vi "ACT_Loop.vi"() -> ()   [LabVIEW 2023, in "Swerve AM_ACT.lvlib"]
uses:
  Swerve AM_ACT.lvlib
  RoboRIO Utilities/Global_STOP.vi
  ENUM_ACT_Action.ctl
  ENUM_ACT_State.ctl
  Global_CMD_ACT_Data In.vi
  Global_ACT_Data Out.vi
  Cluster_CMD_ACT_Data.ctl
  <vilib>/Rock Robotics/WPI/MotorControl/WPI_MotorControlType.ctl
  <vilib>/Rock Robotics/SystemInterfaces/DIO/FPGA_DIOPWMChannel.ctl
  <vilib>/Rock Robotics/WPI/PWM/WPI_PWMDeadband.ctl
  <vilib>/Rock Robotics/SystemInterfaces/DIO/FPGA_DIOChannel.ctl
  <vilib>/Rock Robotics/WPI/MotorControl/WPI_MotorControlDeviceRef.ctl
  <vilib>/Rock Robotics/WPI/ThirdParty/Phoenix-LabVIEW/Motor Controller/Controls/CTRE_Phoenix_MotorControl_NeutralMode.ctl
  Shared Code/TypeDefs/Cluster_FWD  REV Values.ctl
  Shared Code/TypeDefs/Cluster_Config SRX Motor Output.ctl
  Shared Code/TypeDefs/Cluster_PID Gains.ctl
  Shared Code/TypeDefs/Cluster_SRX SLOT PID Config.ctl
  Cluster_Config HW Values.ctl
  b5508d6c-c1cc-4273-80c5-2077d34e1483.vi
  5f725c2a-0ce1-4524-8967-e83b15fdce90.vi
  <vilib>/Rock Robotics/WPI/ThirdParty/Phoenix-LabVIEW/Motor Controller/Controls/CTRE_Phoenix_MotorControl_ControlMode.ctl
  Cluster_HW Output Values.ctl
  ENUM_CMD_Mode Select.ctl
  4f1f8321-3dc8-4b28-8619-20673fc77ec2.vi
  Cluster_System Output Data.ctl
  Cluster_Config System Values.ctl
  36677ea0-a1a5-47a3-bc56-4475cb7c281e.vi
  573e44c0-11f4-4bd9-ad56-904ec25dba75.vi
  e7494af9-f670-4352-9dfa-ae6ce50709ea.vi
  6201c2b1-dcd8-4430-86f1-9b4ee56c7753.vi
  Shared Code/TypeDefs/ENUM_Module Position.ctl
  t-shirt-robot/T-Shirt Robot LV 2020/roboRIO Code/Systems/SwerveDrive AM/Cluster_Config Specific Data.ctl
  t-shirt-robot/T-Shirt Robot LV 2020/roboRIO Code/Systems/SwerveDrive AM/Cluster_Config Specific HW Values.ctl
  Shared Code/TypeDefs/Dial_Compase heading unit circle CCW positive.ctl
  Shared Code/TypeDefs/Level_Velocity plus-minus 1.ctl
  Shared Code/TypeDefs/Cluster_Module Velocity-Direction-Rotations.ctl
  Shared Code/TypeDefs/Cluster_Swerve 4 Steer and Velocity.ctl
  Shared Code/TypeDefs/Cluster_Config_SwerveParam Drive.ctl
  Shared Code/TypeDefs/Cluster_Config_SwerveParam Steer.ctl
  Type Defs/Cluster_Length and Width.ctl
  Cluster_Config Steer HW Values.ctl
  t-shirt-robot/T-Shirt Robot LV 2020/roboRIO Code/Systems/SwerveDrive AM/Cluster_Config Drive HW Values.ctl
  Shared Code/TypeDefs/Cluster_X-Y.ctl
  Shared Code/TypeDefs/Cluster_CMD_Direction Data.ctl
  PigeonIMU/Global_SEN_Data Out.vi
  PigeonIMU/PigeonIMU_SEN_ts.lvlib
  089052c0-d540-4a78-a5cc-aeb70dbb496b.vi
  f366bc00-a3dd-4e55-84f0-76161afbb392.vi
  6826157a-0860-4dcc-86dd-81ceae711a6e.vi
  Shared Code/TypeDefs/Cluster_Config Spark Max Motor Output.ctl
  <vilib>/Rock Robotics/WPI/ThirdParty/REV Robotics/REVLib/Typedef/Spark MAX Idle Mode.ctl
  Shared Code/TypeDefs/Cluster_High-Low.ctl
  Shared Code/TypeDefs/Cluster_Spark MAX SLOT PID Config.ctl
  Shared Code/TypeDefs/Cluster_SW PID Config.ctl
  cae143b2-6fb3-4693-aed3-53517d8ac0dc.vi
  c90b907c-c448-477a-a93b-8b17a70bee0e.vi
  Shared Code/TypeDefs/Cluster_SparkMax Smart Motion Parameters.ctl
  Shared Code/TypeDefs/Cluster_SRX Motion Magic Parameters.ctl
panel:
  in  "Config Drive":T1={"Drive HW Ver"=0, "SparkMax Output"={"Idle Mode"=enum."Coast", "Ramp Rate (S)"=0.0}, "Slot 0 CL"={"Gains"={"P"=0.1, "I"=0.0, "D"=0.0, "F"=0.0}, "I Zone"=0.0, "Peak Out -1 0 1"={"High"=0.0, "Low"=0.0}, "Max I Accu"=0.0}, "Slot 0 SM"={"Max Velocity"=1.0, "Max Acceleration"=0.0, "Allowed CL Error"=0.0, "Min Velocity Output"=0.0}} {"Slot 0 CL"."Gains"."F" format="%#.8f"; "Slot 0 CL"."Gains"."D" format="%#.8f"; "Slot 0 CL"."Gains"."I" format="%#.8f"; "Slot 0 CL"."Gains"."P" format="%#.8f"; "Slot 0 CL"."Peak Out -1 0 1"."Low" format="%#.8f"; "Slot 0 CL"."Peak Out -1 0 1"."High" format="%#.8f"}
  in  "Config Steer":T8={"Steer HW Ver"=0, "SRX Output"={"Neutral"=enum."Override to Coast", "Max"={"FWD"=1.0, "REV"=-1.0}, "Min"={"FWD"=0.0, "REV"=0.0}, "OL Ramp Rate (S)"=0.0, "Dead Band"=0.0, "CL Ramp Rate (S)"=0.0}, "Slot 0 CL"={"Gains"={"P"=1.0, "I"=0.01, "D"=0.0, "F"=0.0}, "Error Allowed"=0.0, "I Zone"=10000.0, "Peak Out 0-1"=1.0, "Max I Accu"=-1000.0}, "Slot 0 MM"={"Cruise Velocity"=5000, "Acceleration"=5000}} {"Slot 0 CL"."Gains"."F" format="%#.8f"; "Slot 0 CL"."Gains"."D" format="%#.8f"; "Slot 0 CL"."Gains"."I" format="%#.8f"; "Slot 0 CL"."Gains"."P" format="%#.8f"; "SRX Output"."Min"."REV" format="%.2f"; "SRX Output"."Min"."FWD" format="%.2f"; "SRX Output"."Max"."REV" format="%.2f"; "SRX Output"."Max"."FWD" format="%.2f"}
  in  "HW Specific Config":T14={"Specific HW Ver"=0, "Specific Data"=[{"Motor Pos"=enum."Left-Front", "CAN Bus"="", "Drive ID"=0, "Drive Invert"=FALSE, "Steer ID"=0, "Steer Invert"=FALSE, "Encoder Start Value"=0.0}, {"Motor Pos"=enum."Right-Front", "CAN Bus"="", "Drive ID"=0, "Drive Invert"=FALSE, "Steer ID"=0, "Steer Invert"=FALSE, "Encoder Start Value"=0.0}, {"Motor Pos"=enum."Right-Back", "CAN Bus"="", "Drive ID"=0, "Drive Invert"=FALSE, "Steer ID"=0, "Steer Invert"=FALSE, "Encoder Start Value"=0.0}, {"Motor Pos"=enum."Left-Back", "CAN Bus"="", "Drive ID"=0, "Drive Invert"=FALSE, "Steer ID"=0, "Steer Invert"=FALSE, "Encoder Start Value"=0.0}]}
  in  "CMD Override":enum32{"None", "Mode 2", "Mode 1", "STOP"}(tab)
  in  "Mode 2 Data":dbl(slide) scale=-0.2..0.2
  in  "Mode 1 Data":i32
  in  "GO":bool
  out "Current Time":timestamp
  in  "System Config":T17={"System Ver"=0, "Auto Angle PID"={"Gains"={"P"=0.1, "I"=0.0, "D"=0.0, "F"=0.0}, "Error Allowed"={"High"=0.0, "Low"=0.0}, "I Zone"={"High"=0.0, "Low"=0.0}, "Peak Out 0-1"={"High"=0.0, "Low"=0.0}, "Max I Accu"={"High"=0.0, "Low"=0.0}}, "Frame"={"Length"=33.0, "Width"=18.0}, "DriveTrain"={"CPR"=14.0, "RevMotor/Wheel"=6.67, "Wheel Diameter (in)"=4.0}, "Speed Full Scale"=5000.0, "Steer Data"={"CPR"=1024.0}} {"Auto Angle PID"."Max I Accu"."Low" format="%#.8f"; "Auto Angle PID"."Max I Accu"."High" format="%#.8f"; "Auto Angle PID"."Gains"."F" format="%#.8f"; "Auto Angle PID"."Gains"."D" format="%#.8f"; "Auto Angle PID"."Gains"."I" format="%#.8f"; "Auto Angle PID"."Gains"."P" format="%#.8f"; "Auto Angle PID"."Error Allowed"."Low" format="%#.8f"; "Auto Angle PID"."Error Allowed"."High" format="%#.8f"; "Auto Angle PID"."I Zone"."Low" format="%#.8f"; "Auto Angle PID"."I Zone"."High" format="%#.8f"; "Auto Angle PID"."Peak Out 0-1"."Low" format="%#.8f"; "Auto Angle PID"."Peak Out 0-1"."High" format="%#.8f"}
  out "System Config":T22
  out "Sensor Read time":dbl format="%.3g"
  out "HW Output":T23 {"Swerve Read"."Back Right"."Angle" scale format="%.3f"; "Swerve Read"."Back Right"."Velocity" scale=-1.0..1.0 scale format="%.1f"; "Swerve Read"."Back Left"."Angle" scale format="%.3f"; "Swerve Read"."Back Left"."Velocity" scale=-1.0..1.0 scale format="%.1f"; "Swerve Read"."Front Left"."Angle" scale format="%.3f"; "Swerve Read"."Front Left"."Velocity" scale=-1.0..1.0 scale format="%.1f"; "Swerve Read"."Front Right"."Angle" scale format="%.3f"; "Swerve Read"."Front Right"."Velocity" scale=-1.0..1.0 scale format="%.1f"; "Pigeon Heading" scale format="%.3f"}
  in  "Read Saved Config":bool
  in  "Update Config":bool
  out "CMD":T28 {"Target Auto Angle" scale format="%.3f"; "Direction"."Rotate(Yaw) CCW 1 CW -1" scale=1.0..-1.0; "Direction"."Traverse"."Angle" scale format="%.3f"; "Direction"."Traverse"."Velocity" scale=-1.0..1.0 scale format="%.1f"}
  out "Cycle Time (S)":dbl format="%.3g"
  # "STOP"
  # "\"Front\" of Robot"
  # "Right Hand Rule"
  # "X"
  # "+CCW"
  # "Y"
  # "(0,0)"
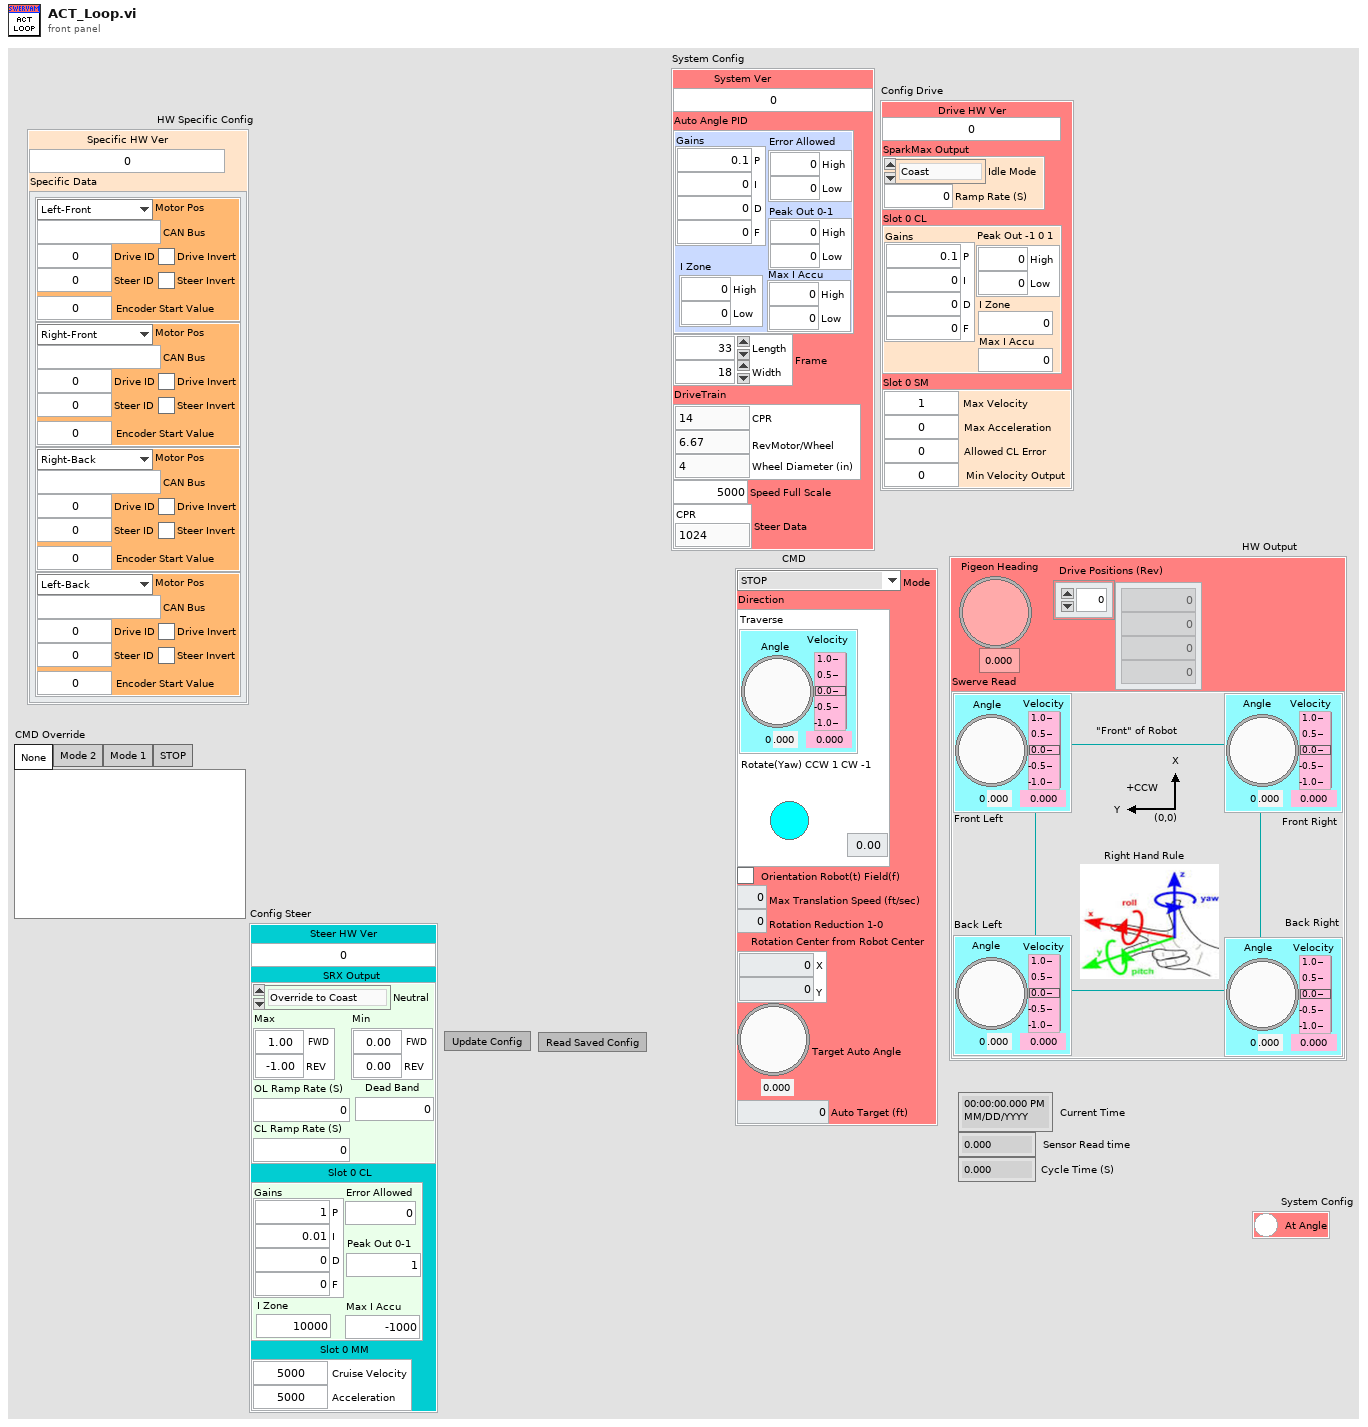
[diagram p1: front panel]
types:
  T1 = typedef "Swerve AM_ACT.lvlib/Cluster_Config Drive HW Values.ctl" = cluster{"Drive HW Ver":u64, "SparkMax Output":T2, "Slot 0 CL":T4, "Slot 0 SM":T7}
  T2 = typedef "Cluster_Config Spark Max Motor Output.ctl" = cluster{"Idle Mode":T3, "Ramp Rate (S)":dbl}
  T3 = typedef "Spark MAX Idle Mode.ctl" = enum16{"Coast", "Brake"}
  T4 = typedef "Cluster_Spark MAX SLOT PID Config.ctl" = cluster{"Gains":T5, "I Zone":dbl, "Peak Out -1 0 1":T6, "Max I Accu":dbl}
  T5 = typedef "Cluster_PID Gains.ctl" = cluster{"P":dbl, "I":dbl, "D":dbl, "F":dbl}
  T6 = typedef "Cluster_High-Low.ctl" = cluster{"High":dbl, "Low":dbl}
  T7 = typedef "Cluster_SparkMax Smart Motion Parameters.ctl" = cluster{"Max Velocity":dbl, "Max Acceleration":dbl, "Allowed CL Error":dbl, "Min Velocity Output":dbl}
  T8 = typedef "Swerve AM_ACT.lvlib/Cluster_Config Steer HW Values.ctl" = cluster{"Steer HW Ver":u64, "SRX Output":T9, "Slot 0 CL":T12, "Slot 0 MM":T13}
  T9 = typedef "Cluster_Config SRX Motor Output.ctl" = cluster{"Neutral":T10, "Max":T11, "Min":T11, "OL Ramp Rate (S)":dbl, "Dead Band":dbl, "CL Ramp Rate (S)":dbl}
  T10 = typedef "CTRE_Phoenix_MotorControl_NeutralMode.ctl" = enum8{"EEPROMSetting", "Override to Coast", "Override to Brake"}
  T11 = typedef "Cluster_FWD  REV Values.ctl" = cluster{"FWD":dbl, "REV":dbl}
  T12 = typedef "Cluster_SRX SLOT PID Config.ctl" = cluster{"Gains":T5, "Error Allowed":dbl, "I Zone":dbl, "Peak Out 0-1":dbl, "Max I Accu":dbl}
  T13 = typedef "Cluster_SRX Motion Magic Parameters.ctl" = cluster{"Cruise Velocity":i32, "Acceleration":i32}
  T14 = typedef "Swerve AM_ACT.lvlib/Cluster_Config Specific HW Values.ctl" = cluster{"Specific HW Ver":u64, "Specific Data":T15[]}
  T15 = typedef "Swerve AM_ACT.lvlib/Cluster_Config Specific Data.ctl" = cluster{"Motor Pos":T16, "CAN Bus":string, "Drive ID":u8, "Drive Invert":bool, "Steer ID":u8, "Steer Invert":bool, "Encoder Start Value":dbl}
  T16 = typedef "ENUM_Module Position.ctl" = enum16{"Left-Front", "Right-Front", "Left-Back", "Right-Back"}
  T17 = typedef "Swerve AM_ACT.lvlib/Cluster_Config System Values.ctl" = cluster{"System Ver":u64, "Auto Angle PID":T18, "Frame":T19, "DriveTrain":T20, "Speed Full Scale":dbl, "Steer Data":T21}
  T18 = typedef "Cluster_SW PID Config.ctl" = cluster{"Gains":T5, "Error Allowed":T6, "I Zone":T6, "Peak Out 0-1":T6, "Max I Accu":T6}
  T19 = typedef "Cluster_Length and Width.ctl" = cluster{"Length":dbl, "Width":dbl}
  T20 = typedef "Cluster_Config_SwerveParam Drive.ctl" = cluster{"CPR":dbl, "RevMotor/Wheel":dbl, "Wheel Diameter (in)":dbl}
  T21 = typedef "Cluster_Config_SwerveParam Steer.ctl" = cluster{"CPR":dbl}
  T22 = typedef "Swerve AM_ACT.lvlib/Cluster_System Output Data.ctl" = cluster{"At Angle":bool}
  T23 = typedef "Swerve AM_ACT.lvlib/Cluster_HW Output Values.ctl" = cluster{"Pigeon Heading":T24, "Swerve Read":T25, "Drive Positions (Rev)":dbl[]}
  T24 = typedef "Dial_Compase heading unit circle CCW positive.ctl" = dbl
  T25 = typedef "Cluster_Swerve 4 Steer and Velocity.ctl" = cluster{"Front Right":T26, "Front Left":T26, "Back Left":T26, "Back Right":T26}
  T26 = typedef "Cluster_Module Velocity-Direction-Rotations.ctl" = cluster{"Velocity":T27, "Angle":T24, "Rotations Count":dbl}
  T27 = typedef "Level_Velocity plus-minus 1.ctl" = dbl
  T28 = typedef "Swerve AM_ACT.lvlib/Cluster_CMD_ACT_Data.ctl" = cluster{"Mode":T29, "Direction":T30, "Orientation Robot(t) Field(f)":bool, "Max Translation Speed (ft/sec)":dbl, "Rotation Reduction 1-0":dbl, "Rotation Center from Robot Center":T31, "Target Auto Angle":T24, "Auto Target (ft)":dbl}
  T29 = typedef "Swerve AM_ACT.lvlib/ENUM_CMD_Mode Select.ctl" = enum16{"STOP", "Move", "Turret Manual", "Trans Manual Angle Auto", "Turret Auto Angle"}
  T30 = typedef "Cluster_CMD_Direction Data.ctl" = cluster{"Traverse":T26, "Rotate(Yaw) CCW 1 CW -1":dbl}
  T31 = typedef "Cluster_X-Y.ctl" = cluster{"X":dbl, "Y":dbl}
  T32 = typedef "Swerve AM_ACT.lvlib/ENUM_ACT_Action.ctl" = enum16{"No Action", "Reset Time", "Reset All", "Config HW File Read", "Config HW File Save", "Config SW File Read", "Config SW File Save", "Config From FP", "Config HW All Get", "Config HW Set Steer", "Open HW Only", "Control FX Stop", "Control FX Mode 1", "Control FX Mode 2", "Set Robot Start Position", "Config HW Set Drive"}
  T33 = typedef "WPI_MotorControlDeviceRef.ctl" = cluster{"DeviceStatus":errorcluster, "Type":T34, "PWM":cluster{"PWM Channel":T35, "DeadBand":T36}, "CAN":cluster{"Device Number":u8, "SetOutput VI Ref":variant, "GetOutput VI Ref":variant, "Enable VI Ref":variant, "Disable VI Ref":variant, "Data":variant}, "Invert":bool, "DIO PWM":cluster{"PWM \"Enable\" Channel":T35, "DIOChannel":T37, "PWM Rate":dbl}}
  T34 = typedef "WPI_MotorControlType.ctl" = enum16{"PWM", "CAN", "DIO PWM"}
  T35 = typedef "FPGA_DIOPWMChannel.ctl" = enum8{"PWM 0", "PWM 1", "PWM 2", "PWM 3", "PWM 4", "PWM 5", "PWM 6", "PWM 7", "PWM 8", "PWM 9", "PWM MXP 0", "PWM MXP 1", "PWM MXP 2", "PWM MXP 3", "PWM MXP 4", "PWM MXP 5", "PWM MXP 6", "PWM MXP 7", "PWM MXP 8", "PWM MXP 9", "Invalid"}
  T36 = typedef "WPI_PWMDeadband.ctl" = cluster{"Name":string, "maxPositivePwm":i32, "minPositivePwm":i32, "centerPwm":i32, "maxNegativePwm":i32, "minNegativePwm":i32, "angularRange":u16}
  T37 = typedef "FPGA_DIOChannel.ctl" = enum8{"DIO 0", "DIO 1", "DIO 2", "DIO 3", "DIO 4", "DIO 5", "DIO 6", "DIO 7", "DIO 8", "DIO 9", "DIO MXP 0", "DIO MXP 1", "DIO MXP 2", "DIO MXP 3", "DIO MXP 4", "DIO MXP 5", "DIO MXP 6", "DIO MXP 7", "DIO MXP 8", "DIO MXP 9", "DIO MXP 10", "DIO MXP 11", "DIO MXP 12", "DIO MXP 13", "DIO MXP 14", "DIO MXP 15", "SPI Port CS1", "SPI Port CS2", "SPI Port CS3", "SPI Port MISO", "SPI Port MOSI", "Invalid"}
  T38 = typedef "Swerve AM_ACT.lvlib/Cluster_Config HW Values.ctl" = cluster{"Drive":T1, "Steer":T8}
  T39 = typedef "CTRE_Phoenix_MotorControl_ControlMode.ctl" = u16
  T40 = typedef "Swerve AM_ACT.lvlib/ENUM_ACT_State.ctl" = enum16{"Startup", "Configuring", "Stopping", "Moving Mode 1", "Moving Mode 2", "Shutdown", "Initializing HW"}
  T41 = cluster{"Motor List":T16[], "Team Folder":path, "FX Ref":T33, "Steer Refs":T33[], "Drive Refs":T33[], "State":T40, "Previous State":T40, "Current Time":timestamp, "Previous Time":timestamp, "Start Time":timestamp, "Target Time (ms)":u32, "Cycle Time(S)":dbl, "Update Display":bool, "ACT Input":T28, "HW All Config":T38, "Config System":T17, "Max # Of Config Tries":i32, "HW Out":T23, "System Output":T22, "CAN Timeout":u32, "FX Mode":T39, "FX Set Value":dbl, "Config HW Specific":T14, "Swerve Set":T25, "New Cmd":bool, "Config HW Steer":T8, "Config HW Drive":T1}
  T42 = enum16{"No Action", "Reset Time", "Reset All", "Config HW File Read", "Config HW File Save", "Config SW File Read", "Config SW File Save", "Config From FP", "Config HW All Get", "Config HW Set Steer", "Open HW Only", "Control FX Stop", "Control FX Mode 1", "Control FX Mode 2", "Set Robot Start Position", "Config HW Set Drive"}
  T43 = cluster{"[0]":T26, "[1]":T26, "[2]":T26, "[3]":T26}
  T44 = typedef "Cluster_Unity Yaw-Pitch-Roll.ctl" = cluster{"Yaw":T24, "Pitch":T24, "Roll":T24}
  T45 = typedef "Swerve AM_ACT.lvlib/ENUM_ACT_Action.ctl" = enum16{"No Action", "Reset Time", "Reset All", "Open HW References", "Control FX Stop", "Control FX Mode 1", "Control FX Mode 2", "Set Robot Start Position", "Config HW Steer Set", "Config HW Steer Get", "Config HW Steer Save", "Config HW Steer Read", "Config HW Drive Set", "Config HW Drive Get", "Config HW Drive Save", "Config HW Drive Read", "Config HW Specific Set", "Config HW Specific Get", "Config HW Specific Save", "Config HW Specific Read", "Config System Save", "Config System Read", "Config From FP", "Start HW Steer Set", "Default HW Steer Set", "Defalut HW Drive Set"}
  T46 = enum16{"No Action", "Reset Time", "Reset All", "Config HW File Read", "Config HW File Save", "Config SW File Read", "Config SW File Save", "Config From FP", "Config HW All Get", "Config HW Set Steer", "Open HW Only", "Control FX Stop", "Control FX Mode 1", "Control FX Mode 2", "Set Robot Start Position", "Config HW Set Drive"}[]
  T47 = typedef "Swerve AM_ACT.lvlib/Cluster_Config HW Values.ctl" = cluster{"Drive":T48, "Steer":T52}
  T48 = typedef "Swerve AM_ACT.lvlib/Cluster_Config Drive Module Values.ctl" = cluster{"Drive HW Ver":u64, "SparkMax Output":T49, "Slot 0 CL":T51}
  T49 = typedef "Cluster_Config Spark Max Motor Output.ctl" = cluster{"Motor Type":T50, "Inverted":bool, "Idle Mode":T3, "OL Ramp Rate (S)":dbl, "CL Ramp Rate (S)":dbl}
  T50 = typedef "Spark MAX Motor Type.ctl" = enum16{"Brushed", "Brushless"}
  T51 = typedef "Cluster_Spark MAX SLOT PID Config.ctl" = cluster{"Gains":T5, "Error Allowed":dbl, "I Zone":dbl, "Peak Out -1 0 1":T6, "Max I Accu":dbl}
  T52 = typedef "Swerve AM_ACT.lvlib/Cluster_Config Steer HW Values.ctl" = cluster{"Steer HW Ver":u64, "SRX Output":T53, "Slot 0 CL":T12, "MM":T13}
  T53 = typedef "Cluster_Config SRX Motor Output.ctl" = cluster{"Inverted":bool, "Neutral":T10, "Max":T11, "Min":T11, "OL Ramp Rate (S)":dbl, "Dead Band":dbl, "CL Ramp Rate (S)":dbl}
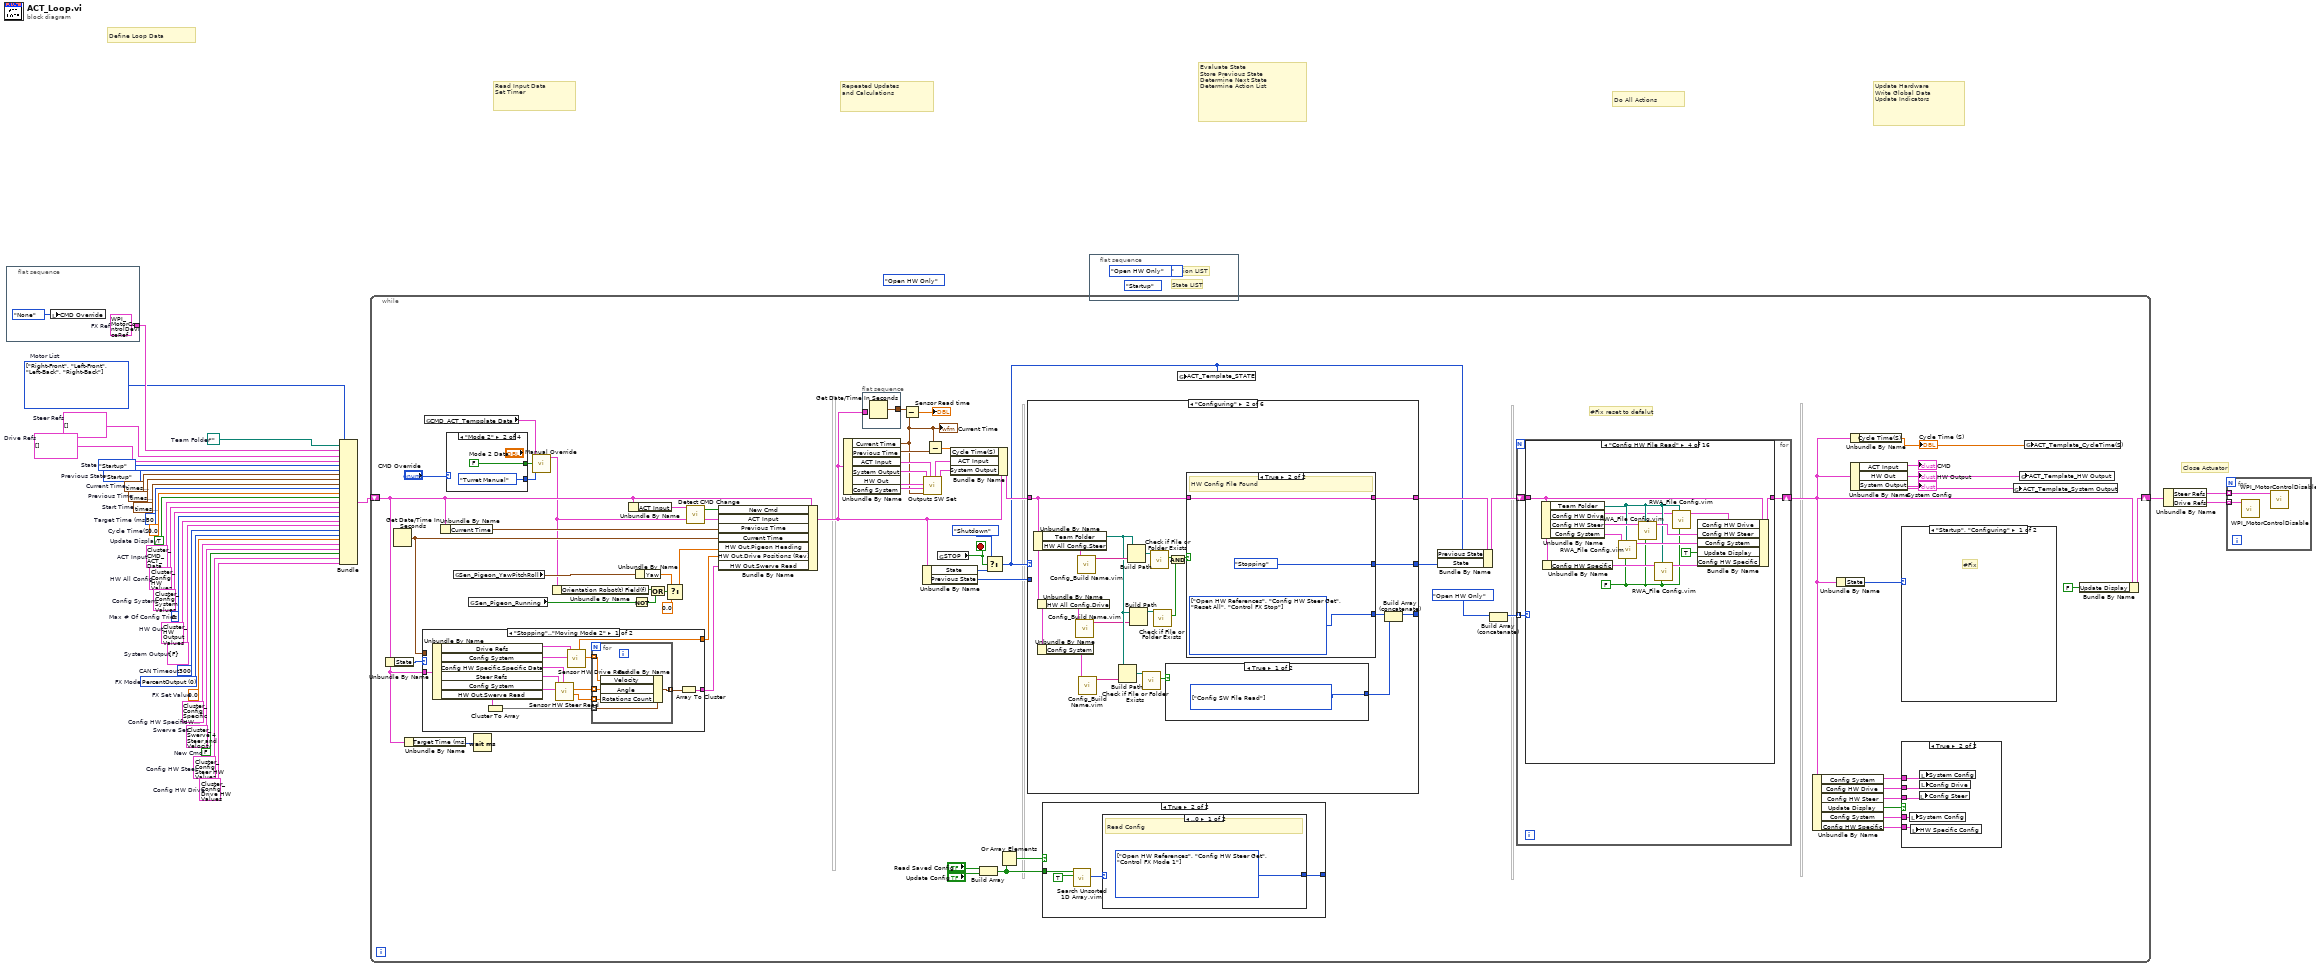
[diagram p0: block diagram]
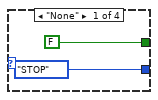
[diagram p2: hidden frame]
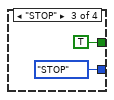
[diagram p3: hidden frame]
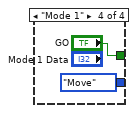
[diagram p4: hidden frame]
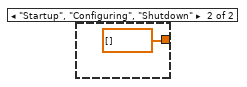
[diagram p5: hidden frame]
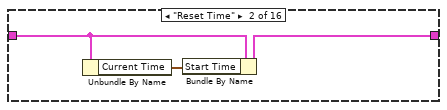
[diagram p7: hidden frame]
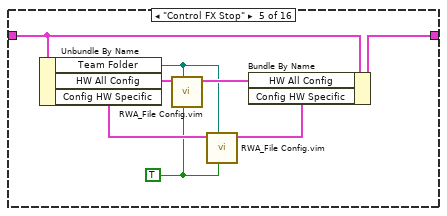
[diagram p9: hidden frame]
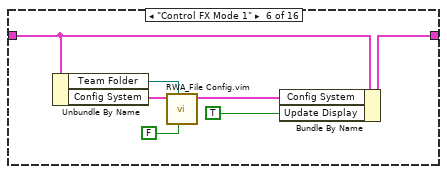
[diagram p10: hidden frame]
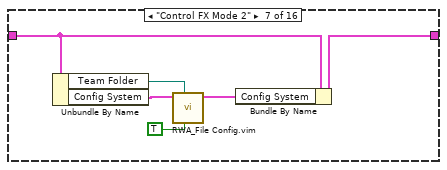
[diagram p11: hidden frame]
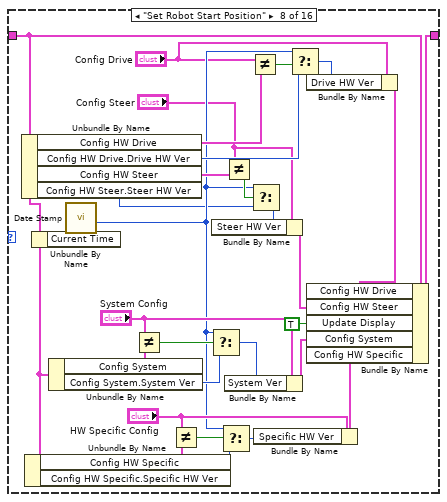
[diagram p12: hidden frame]
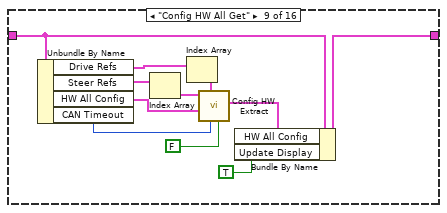
[diagram p13: hidden frame]
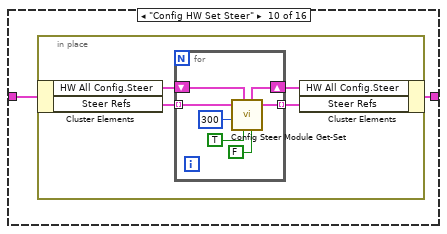
[diagram p14: hidden frame]
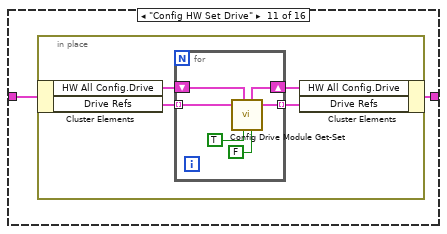
[diagram p15: hidden frame]
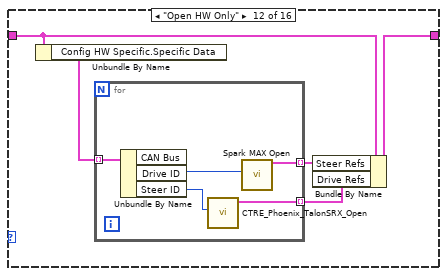
[diagram p16: hidden frame]
diagram:
  (unwired) ENUM_ACT_Action."Open HW Only" ("Action")
  w2 = T8 {"Steer HW Ver"=0, "SRX Output"={"Neutral"=enum."Override to Coast", "Max"={"FWD"=1.0, "REV"=-1.0}, "Min"={"FWD"=0.0, "REV"=0.0}, "OL Ramp Rate (S)"=0.0, "Dead Band"=0.0, "CL Ramp Rate (S)"=0.0}, "Slot 0 CL"={"Gains"={"P"=1.0, "I"=0.01, "D"=0.0, "F"=0.0}, "Error Allowed"=0.0, "I Zone"=10000.0, "Peak Out 0-1"=1.0, "Max I Accu"=-1000.0}, "Slot 0 MM"={"Cruise Velocity"=5000, "Acceleration"=5000}}  # Config HW Steer
  w1 = T1 {"Drive HW Ver"=0, "SparkMax Output"={"Idle Mode"=enum."Coast", "Ramp Rate (S)"=0.0}, "Slot 0 CL"={"Gains"={"P"=0.1, "I"=0.0, "D"=0.0, "F"=0.0}, "I Zone"=0.0, "Peak Out -1 0 1"={"High"=0.0, "Low"=0.0}, "Max I Accu"=0.0}, "Slot 0 SM"={"Max Velocity"=1.0, "Max Acceleration"=0.0, "Allowed CL Error"=0.0, "Min Velocity Output"=0.0}}  # Config HW Drive
  w3 = FALSE  # New Cmd
  w4 = path ""  # Team Folder
  w6 = T25 {"Front Right"={"Velocity"=0.0, "Angle"=0.0, "Rotations Count"=0.0}, "Front Left"={"Velocity"=0.0, "Angle"=0.0, "Rotations Count"=0.0}, "Back Left"={"Velocity"=0.0, "Angle"=0.0, "Rotations Count"=0.0}, "Back Right"={"Velocity"=0.0, "Angle"=0.0, "Rotations Count"=0.0}}  # Swerve Set
  w7 = T16[] [enum."Right-Front", enum."Left-Front", enum."Left-Back", enum."Right-Back"] items=["Left-Front", "Right-Front", "Left-Back", "Right-Back"]  # Motor List
  w10 = T33[] []  # Steer Refs
  w9 = T33[] []  # Drive Refs
  w11 = T14 {"Specific HW Ver"=0, "Specific Data"=[{"Motor Pos"=enum."Left-Front", "CAN Bus"="", "Drive ID"=0, "Drive Invert"=FALSE, "Steer ID"=0, "Steer Invert"=FALSE, "Encoder Start Value"=0.0}, {"Motor Pos"=enum."Right-Front", "CAN Bus"="", "Drive ID"=0, "Drive Invert"=FALSE, "Steer ID"=0, "Steer Invert"=FALSE, "Encoder Start Value"=0.0}, {"Motor Pos"=enum."Right-Back", "CAN Bus"="", "Drive ID"=0, "Drive Invert"=FALSE, "Steer ID"=0, "Steer Invert"=FALSE, "Encoder Start Value"=0.0}, {"Motor Pos"=enum."Left-Back", "CAN Bus"="", "Drive ID"=0, "Drive Invert"=FALSE, "Steer ID"=0, "Steer Invert"=FALSE, "Encoder Start Value"=0.0}]}  # Config HW Specific
  w20 = T38 {"Drive"={"Drive HW Ver"=0, "SparkMax Output"={"Idle Mode"=enum."Coast", "Ramp Rate (S)"=0.0}, "Slot 0 CL"={"Gains"={"P"=0.0, "I"=0.0, "D"=0.0, "F"=0.0}, "I Zone"=0.0, "Peak Out -1 0 1"={"High"=0.0, "Low"=0.0}, "Max I Accu"=0.0}, "Slot 0 SM"={"Max Velocity"=0.0, "Max Acceleration"=0.0, "Allowed CL Error"=0.0, "Min Velocity Output"=0.0}}, "Steer"={"Steer HW Ver"=0, "SRX Output"={"Neutral"=enum."Override to Coast", "Max"={"FWD"=1.0, "REV"=-1.0}, "Min"={"FWD"=0.0, "REV"=0.0}, "OL Ramp Rate (S)"=0.0, "Dead Band"=0.0, "CL Ramp Rate (S)"=0.0}, "Slot 0 CL"={"Gains"={"P"=1.0, "I"=0.01, "D"=0.0, "F"=0.0}, "Error Allowed"=0.0, "I Zone"=10.0, "Peak Out 0-1"=1.0, "Max I Accu"=-10.0}, "Slot 0 MM"={"Cruise Velocity"=5000, "Acceleration"=5000}}}  # HW All Config
  w17 = T22 {"At Angle"=FALSE}  # System Output
  w19 = T17 {"System Ver"=0, "Auto Angle PID"={"Gains"={"P"=0.2, "I"=0.0, "D"=0.0, "F"=0.0}, "Error Allowed"={"High"=0.0, "Low"=0.0}, "I Zone"={"High"=0.0, "Low"=0.0}, "Peak Out 0-1"={"High"=0.0, "Low"=0.0}, "Max I Accu"={"High"=0.0, "Low"=0.0}}, "Frame"={"Length"=33.0, "Width"=18.0}, "DriveTrain"={"CPR"=14.0, "RevMotor/Wheel"=6.67, "Wheel Diameter (in)"=4.0}, "Speed Full Scale"=5000.0, "Steer Data"={"CPR"=1024.0}}  # Config System
  w18 = T23 {"Pigeon Heading"=0.0, "Swerve Read"={"Front Right"={"Velocity"=0.0, "Angle"=0.0, "Rotations Count"=0.0}, "Front Left"={"Velocity"=0.0, "Angle"=0.0, "Rotations Count"=0.0}, "Back Left"={"Velocity"=0.0, "Angle"=0.0, "Rotations Count"=0.0}, "Back Right"={"Velocity"=0.0, "Angle"=0.0, "Rotations Count"=0.0}}, "Drive Positions (Rev)"=[]}  # HW Out
  w14 = 0.0  # FX Set Value
  w15 = T39 0 items=["PercentOutput"=0, "Position"=1, "Velocity"=2, "Current"=3, "Follower"=5, "MotionProfile"=6, "MotionMagic"=7, "MotionProfileArc"=10, "Disabled"=15]  # FX Mode
  w13 = u32 300  # CAN Timeout
  w12 = 3  # Max # Of Config Tries
  w22 = TRUE  # Update Display
  w25 = 0.0  # Cycle Time(S)
  w26 = ENUM_ACT_State."Startup"  # Previous State
  w27 = timestamp(0 s since 1904-01-01)  # Previous Time
  w28 = u32 50  # Target Time (ms)
  w16 = T28 {"Mode"=enum."STOP", "Direction"={"Traverse"={"Velocity"=0.0, "Angle"=0.0, "Rotations Count"=0.0}, "Rotate(Yaw) CCW 1 CW -1"=0.0}, "Orientation Robot(t) Field(f)"=FALSE, "Max Translation Speed (ft/sec)"=0.0, "Rotation Reduction 1-0"=0.0, "Rotation Center from Robot Center"={"X"=0.0, "Y"=0.0}, "Target Auto Angle"=0.0, "Auto Target (ft)"=0.0}  # ACT Input
  w29 = timestamp(0 s since 1904-01-01)  # Start Time
  w30 = timestamp(0 s since 1904-01-01)  # Current Time
  w31 = ENUM_ACT_State."Startup"  # State
  # "Close Actuator"
  # "Define Loop Data"
  # "Repeated Updates\nand Calculations"
  # "Read Input Data\nSet Timer"
  # "Evaluate State\nStore Previous State\nDetermine Next State\nDetermine Action List"
  # "Do All Actions"
  # "Update Hardware\nWrite Global Data\nUpdate Indicators"
  n1 = flat-sequence {
    tunnel: [w33] -> w23
    frame #0 {
      w33 = T33 {"DeviceStatus"={"status"=FALSE, "code"=0, "source"=""}, "Type"=enum."PWM", "PWM"={"PWM Channel"=enum."PWM 1", "DeadBand"={"Name"="", "maxPositivePwm"=0, "minPositivePwm"=0, "centerPwm"=0, "maxNegativePwm"=0, "minNegativePwm"=0, "angularRange"=0}}, "CAN"={"Device Number"=0, "SetOutput VI Ref"=variant(enum8{"Percent VBus", "Current", "Speed", "Position", "Voltage"} enum."Percent VBus"), "GetOutput VI Ref"=variant(refnum<k1> refnum), "Enable VI Ref"=variant(dbl 12.0), "Disable VI Ref"=variant(enum8{"Percent VBus", "Speed", "Position", "Slave", "Unchanged / Invalid", "Voltage Compensation", "Current", "Motion Profile"} enum."Percent VBus"), "Data"=variant}, "Invert"=FALSE, "DIO PWM"={"PWM \"Enable\" Channel"=enum."Invalid", "DIOChannel"=enum."Invalid", "PWM Rate"=0.0}}  # FX Ref
      n2 = local write "CMD Override"(enum32{"None", "Mode 2", "Mode 1", "STOP"}."None" ("CMD Override")) -> ()
    }
  }
  n3 = Bundle("Motor List"=w7, "Team Folder"=w4, "FX Ref"=w23, "Steer Refs"=w10, "Drive Refs"=w9, "State"=w31, "Previous State"=w26, "Current Time"=w30, "Previous Time"=w27, "Start Time"=w29, "Target Time (ms)"=w28, "Cycle Time(S)"=w25, "Update Display"=w22, "ACT Input"=w16, "HW All Config"=w20, "Config System"=w19, "Max # Of Config Tries"=w12, "HW Out"=w18, "System Output"=w17, "CAN Timeout"=w13, "FX Mode"=w15, "FX Set Value"=w14, "Config HW Specific"=w11, "Swerve Set"=w6, "New Cmd"=w3, "Config HW Steer"=w2, "Config HW Drive"=w1) -> (w5:T41)  [unwired: 1 in]
  n4 = while {
    shift-right: [w84] -> w24
    shift-left: w5 -> [w41]
    stop <- w94 stop-if-true
    # "#Fix reset to defalut"
    n5 = Unbundle By Name(w41) -> ("State"=w76:T40)
    n6 = Get Date/Time In Seconds() -> (seconds since 1Jan1904=w72:timestamp)
    n7 = Unbundle By Name(w41) -> ("Target Time (ms)"=w91:u32)
    n8 = case shown="\"Stopping\"..\"Moving Mode 2\"" w76 {
      tunnel: w41 -> [w118 _]
      tunnel: w72 -> [_ _]
      tunnel: [w113 _] -> w42
      tunnel: [w108 dbl[] [] ("Drive Positions (Rev) Out")] -> w43
      frame "Stopping".."Moving Mode 2" {
        n9 = Unbundle By Name(w118) -> ("Drive Refs"=w119:T33[], "Config System"=w116:T17, "Config HW Specific.Specific Data"=w117:T15[], "Steer Refs"=w120:T33[], "Config System"=w107:T17, "HW Out.Swerve Read"=w115:T25)
        n10 = Cluster To Array(cluster=w115) -> (array=w114:T26[])
        n11 = call "Sensor HW Steer Read.vi"("HW Specific Config.Specific Data"=w117, "Steer"=w107, "Steer Ref"=w120) -> ("Offsets Out"=w109:dbl[], "Angles Out"=w110:dbl[])  [unwired: 5 in, 2 out]
        n12 = call "Sensor HW Drive Read.vi"("Config HW Drive Values"=w116, "Drive Ref"=w119) -> ("Drive Velocities (0-1) Out"=w111:dbl[], "Drive Positions (Rev) Out"=w108:dbl[])  [unwired: 6 in, 2 out]
        n13 = for {
          tunnel: w114 -> [w125] mode=indexing
          tunnel: [w124] -> w112 mode=indexing
          tunnel: w111 -> [w123] mode=indexing
          tunnel: w110 -> [w122] mode=indexing
          tunnel: w109 -> [w121] mode=indexing
          n14 = Bundle By Name(cluster=w125, "Velocity"=w123, "Angle"=w122, "Rotations Count"=w121) -> (w124:T26)
        }
        n15 = Array To Cluster(array=w112) -> (cluster=w113:T43)
      }
      frame "Startup", "Configuring", "Shutdown" {
      }
    }
    n16 = global read "Global_CMD_ACT_Data In.vi" "CMD_ACT_Tempplate Data"() -> (w48:T28)
    n17 = Unbundle By Name(w41) -> ("Current Time"=w90:timestamp)
    n18 = case shown="\"Mode 2\"" "CMD Override" {
      tunnel: [FALSE ("Enable") FALSE ("Enable") TRUE ("Positon GO") "GO"] -> w58
      tunnel: [ENUM_CMD_Mode_Select."STOP" ("Override") ENUM_CMD_Mode_Select."Turret Manual" ("Override") ENUM_CMD_Mode_Select."STOP" ("Override") ENUM_CMD_Mode_Select."Move" ("Override")] -> w57
      frame "None" {
      }
      frame "Mode 2" {
      }
      frame "STOP" {
      }
      frame "Mode 1" {
      }
    }
    n19 = global read "Global_SEN_Data Out.vi" "Sen_Pigeon_YawPitchRoll"() -> (w54:T44)
    n20 = global read "Global_SEN_Data Out.vi" "Sen_Pigeon_Running"() -> (w51:bool)
    n21 = Wait (ms)(milliseconds to wait=w91) -> ()  [unwired: 1 out]
    n22 = call "Manual Override.vi"("Override"=w57, "Enable"=w58, "Auto CMD"=w48) -> ("OverRide Command Out"=w39:T28)  [unwired: 8 in]
    n23 = Unbundle By Name(w39) -> ("Orientation Robot(t) Field(f)"=w55:bool)
    n24 = Unbundle By Name(w41) -> ("ACT Input"=w40:T28)
    n25 = Not(x=w51) -> (.not. x?=w50:bool)
    n26 = Unbundle By Name(w54) -> ("Yaw"=w49:T24)
    n27 = Or(x=w55, y=w50) -> (x .or. y?=w52:bool)
    n28 = Select(t=T24 0.0, s=w52, f=w49) -> (s? t:f=w47:T24)
    n29 = call "Detect CMD Change.vi"("CMD_ACT_SwerveDrive_Data"=w39, "Preious ACT Input"=w40) -> ("New Command"=w38:bool)  [unwired: 9 in]
    n30 = Bundle By Name(cluster=w41, "New Cmd"=w38, "ACT Input"=w39, "Previous Time"=w90, "Current Time"=w72, "HW Out.Pigeon Heading"=w47, "HW Out.Drive Positions (Rev)"=w43, "HW Out.Swerve Read"=w42) -> (w60:T41)
    n31 = Unbundle By Name(w60) -> ("Current Time"=w35:timestamp, "Previous Time"=w88:timestamp, "ACT Input"=w46:T28, "System Output"=w65:T22, "HW Out"=w63:T23, "Config System"=w62:T17)
    "Current Time" <- w35
    n32 = flat-sequence {
      tunnel: [w106] -> w74
      tunnel: w60 -> [_]
      frame #0 {
        n33 = Get Date/Time In Seconds() -> (seconds since 1Jan1904=w106:timestamp)
      }
    }
    n34 = Subtract(x=w74, y=w35) -> (x-y=→"Sensor Read time":dbl)
    n35 = Unbundle By Name(w60) -> ("State"=w92:T40, "Previous State"=w89:T40)
    n36 = call "Outputs SW Set.vi"("Auto CMD"=w46, "Current Time"=w35, "System Config"=w62, "Sensor Values"=w63, "SW Output"=w65) -> ("SW Output Out"=w64:T22, "Auto CMD Out"=w45:T28)  [unwired: 5 in]
    n37 = Subtract(x=w35, y=w88) -> (x-y=w86:dbl)
    n38 = global read "Global_STOP.vi" "STOP"() -> (w94:bool)
    n39 = Bundle By Name(cluster=w60, "Cycle Time(S)"=w86, "ACT Input"=w45, "System Output"=w64) -> (w87:T41)
    n40 = Build Array("Read Saved Config", "Update Config") -> (w68:bool[])
    n41 = Select(t=ENUM_ACT_State."Shutdown" ("State"), s=w94, f=w92) -> (s? t:f=w56:T40)
    n42 = Or Array Elements(Boolean array=w68) -> (logical OR=w69:bool)
    n43 = case shown="\"Configuring\"" w56 {
      selector: w56 -> [_ _ _ w308 w330 _]
      tunnel: w87 -> [w253 w267 w289 w309 w331 w352]
      tunnel: [w254 w272 w288 w310 w332 w352] -> w96
      tunnel: [ENUM_ACT_State."Configuring" ("State") w271 w287 w312 w334 ENUM_ACT_State."Shutdown" ("State")] -> w95
      tunnel: [w256 w257 w285 w307 w328 w350] -> _
      tunnel: w89 -> [_ _ _ _ _ _]
      frame "Startup" {
        w256 = T45[] [enum."Reset Time"] items=["No Action", "Reset Time", "Reset All", "Open HW References", "Control FX Stop", "Control FX Mode 1", "Control FX Mode 2", "Set Robot Start Position", "Config HW Steer Set", "Config HW Steer Get", "Config HW Steer Save", "Config HW Steer Read", "Config HW Drive Set", "Config HW Drive Get", "Config HW Drive Save", "Config HW Drive Read", "Config HW Specific Set", "Config HW Specific Get", "Config HW Specific Save", "Config HW Specific Read", "Config System Save", "Config System Read", "Config From FP", "Start HW Steer Set", "Default HW Steer Set", "Defalut HW Drive Set"] ("Actions")
        n44 = call "File RIO_Get or Create Team Folder.vi"() -> ("Team Files Folder"=w252:path)  [unwired: 10 in, 1 out]
        n45 = call "Config Default.vi"() -> ("System Config Out"=w248:T17, "Drive Default Out"=w249:T1, "Steer Default Out"=w250:T8, "Module Specific Default Out"=w251:T14)  [unwired: 8 in]
        n46 = Bundle By Name(cluster=w253, "Team Folder"=w252, "Config HW Specific"=w251, "HW All Config.Steer"=w250, "HW All Config.Drive"=w249, "Config System"=w248) -> (w254:T41)
      }
      frame "Configuring" {
        n47 = Unbundle By Name(w267) -> ("Team Folder"=w264:path, "HW All Config.Steer"=w274:T8)
        n48 = Unbundle By Name(w267) -> ("HW All Config.Drive"=w265:T1)
        n49 = Unbundle By Name(w267) -> ("Config System"=w269:T17)
        n50 = call "Config_Build Name.vim"("Config First Name"=w265) -> ("Cfg file"=w263:string)  [unwired: 9 in, 1 out]
        n51 = call "Config_Build Name.vim"("Config First Name"=w274) -> ("Cfg file"=w276:string)  [unwired: 9 in, 1 out]
        n52 = call "Config_Build Name.vim"("Config First Name"=w269) -> ("Cfg file"=w270:string)  [unwired: 9 in, 1 out]
        n53 = Build Path(base path=w264, name or relative path=w270) -> (appended path=w268:path)
        n54 = Build Path(base path=w264, name or relative path=w276) -> (appended path=w275:path)
        n55 = Build Path(base path=w264, name or relative path=w263) -> (appended path=w262:path)
        n56 = call <vilib>:"Check if File or Folder Exists.vi"("path"=w268) -> ("file or folder exists?"=w260:bool)  [unwired: 8 in, 2 out]
        n57 = call <vilib>:"Check if File or Folder Exists.vi"("path"=w275) -> ("file or folder exists?"=w273:bool)  [unwired: 8 in, 2 out]
        n58 = call <vilib>:"Check if File or Folder Exists.vi"("path"=w262) -> ("file or folder exists?"=w261:bool)  [unwired: 8 in, 2 out]
        n59 = case shown="True" w260 {
          tunnel: [w277 w278] -> w259
          frame True {
            w277 = T32[] [enum."Config SW File Read"] items=["No Action", "Reset Time", "Reset All", "Config HW File Read", "Config HW File Save", "Config SW File Read", "Config SW File Save", "Config From FP", "Config HW All Get", "Config HW Set Steer", "Open HW Only", "Control FX Stop", "Control FX Mode 1", "Control FX Mode 2", "Set Robot Start Position", "Config HW Set Drive"] ("Actions")
          }
          frame False {
            w278 = T45[] [enum."Control FX Mode 2"] items=["No Action", "Reset Time", "Reset All", "Open HW References", "Control FX Stop", "Control FX Mode 1", "Control FX Mode 2", "Set Robot Start Position", "Config HW Steer Set", "Config HW Steer Get", "Config HW Steer Save", "Config HW Steer Read", "Config HW Drive Set", "Config HW Drive Get", "Config HW Drive Save", "Config HW Drive Read", "Config HW Specific Set", "Config HW Specific Get", "Config HW Specific Save", "Config HW Specific Read", "Config System Save", "Config System Read", "Config From FP", "Start HW Steer Set", "Default HW Steer Set", "Defalut HW Drive Set"] ("Actions")
          }
        }
        n60 = And(x=w273, y=w261) -> (x .and. y?=w266:bool)
        n61 = case shown="True" w266 {
          tunnel: w267 -> [w281 w284]
          tunnel: [w281 w284] -> w272
          tunnel: [ENUM_ACT_State."Configuring" ("State") ENUM_ACT_State."Stopping" ("State")] -> w271
          tunnel: [w279 w282] -> w258
          frame False {
            w279 = T32[] [enum."Open HW Only", enum."Config HW All Get", enum."Config HW File Save"] items=["No Action", "Reset Time", "Reset All", "Config HW File Read", "Config HW File Save", "Config SW File Read", "Config SW File Save", "Config From FP", "Config HW All Get", "Config HW Set Steer", "Open HW Only", "Control FX Stop", "Control FX Mode 1", "Control FX Mode 2", "Set Robot Start Position", "Config HW Set Drive"] ("Actions")
            # "HW Config File Not Found"
          }
          frame True {
            w282 = T45[] [enum."Open HW References", enum."Config HW Steer Get", enum."Reset All", enum."Control FX Stop"] items=["No Action", "Reset Time", "Reset All", "Open HW References", "Control FX Stop", "Control FX Mode 1", "Control FX Mode 2", "Set Robot Start Position", "Config HW Steer Set", "Config HW Steer Get", "Config HW Steer Save", "Config HW Steer Read", "Config HW Drive Set", "Config HW Drive Get", "Config HW Drive Save", "Config HW Drive Read", "Config HW Specific Set", "Config HW Specific Get", "Config HW Specific Save", "Config HW Specific Read", "Config System Save", "Config System Read", "Config From FP", "Start HW Steer Set", "Default HW Steer Set", "Defalut HW Drive Set"] ("Actions")
            # "HW Config File Found"
          }
        }
        n62 = Build Array (concatenate)(w258, w259) -> (w257:u16[])
      }
      frame "Stopping" {
        (unwired) TRUE
        w286 = T45[] [enum."Control FX Stop"] items=["No Action", "Reset Time", "Reset All", "Open HW References", "Control FX Stop", "Control FX Mode 1", "Control FX Mode 2", "Set Robot Start Position", "Config HW Steer Set", "Config HW Steer Get", "Config HW Steer Save", "Config HW Steer Read", "Config HW Drive Set", "Config HW Drive Get", "Config HW Drive Save", "Config HW Drive Read", "Config HW Specific Set", "Config HW Specific Get", "Config HW Specific Save", "Config HW Specific Read", "Config System Save", "Config System Read", "Config From FP", "Start HW Steer Set", "Default HW Steer Set", "Defalut HW Drive Set"] ("Actions")
        n63 = Unbundle By Name(w289) -> ("ACT Input.Mode"=w290:T29)
        n64 = case shown="\"Turret Auto Angle\"" w290 {
          tunnel: w289 -> [w293 w296 w299 w302 w305]
          tunnel: [w293 w296 w299 w302 w305] -> w288
          tunnel: [ENUM_ACT_State."Stopping" ("State") ENUM_ACT_State."Moving Mode 1" ("State") ENUM_ACT_State."Moving Mode 2" ("State") ENUM_ACT_State."Moving Mode 2" ("State") ENUM_ACT_State."Moving Mode 2" ("State")] -> w287
          tunnel: [w291 w294 w297 w300 w303] -> w285
          tunnel: w286 -> [w291 w294 w297 w300 w303]
          frame "STOP" {
          }
          frame "Move" {
          }
          frame "Turret Manual" {
          }
          frame "Trans Manual Angle Auto" {
          }
          frame "Turret Auto Angle" {
          }
        }
      }
      frame "Moving Mode 1" {
        w306 = T45[] [enum."Control FX Stop"] items=["No Action", "Reset Time", "Reset All", "Open HW References", "Control FX Stop", "Control FX Mode 1", "Control FX Mode 2", "Set Robot Start Position", "Config HW Steer Set", "Config HW Steer Get", "Config HW Steer Save", "Config HW Steer Read", "Config HW Drive Set", "Config HW Drive Get", "Config HW Drive Save", "Config HW Drive Read", "Config HW Specific Set", "Config HW Specific Get", "Config HW Specific Save", "Config HW Specific Read", "Config System Save", "Config System Read", "Config From FP", "Start HW Steer Set", "Default HW Steer Set", "Defalut HW Drive Set"] ("Actions")
        n65 = Unbundle By Name(w309) -> ("ACT Input.Mode"=w311:T29)
        n66 = case shown="\"Turret Auto Angle\"" w311 {
          tunnel: [ENUM_ACT_State."Stopping" ("State") ENUM_ACT_State."Moving Mode 2" ("State") ENUM_ACT_State."Moving Mode 2" ("State") ENUM_ACT_State."Moving Mode 2" ("State") w326] -> w312
          tunnel: w309 -> [w315 w318 w321 w324 w327]
          tunnel: [w315 w318 w321 w324 w327] -> w310
          tunnel: w308 -> [_ _ _ _ w326]
          tunnel: [w313 w316 w319 w322 w325] -> w307
          tunnel: w306 -> [w313 w316 w319 w322 _]
          frame "STOP" {
          }
          frame "Turret Manual" {
          }
          frame "Trans Manual Angle Auto" {
          }
          frame "Turret Auto Angle" {
          }
          frame "Move" {
            w325 = T45[] [enum."Control FX Mode 1"] items=["No Action", "Reset Time", "Reset All", "Open HW References", "Control FX Stop", "Control FX Mode 1", "Control FX Mode 2", "Set Robot Start Position", "Config HW Steer Set", "Config HW Steer Get", "Config HW Steer Save", "Config HW Steer Read", "Config HW Drive Set", "Config HW Drive Get", "Config HW Drive Save", "Config HW Drive Read", "Config HW Specific Set", "Config HW Specific Get", "Config HW Specific Save", "Config HW Specific Read", "Config System Save", "Config System Read", "Config From FP", "Start HW Steer Set", "Default HW Steer Set", "Defalut HW Drive Set"] ("Actions")
          }
        }
      }
      frame "Moving Mode 2" {
        w329 = T45[] [enum."Control FX Stop"] items=["No Action", "Reset Time", "Reset All", "Open HW References", "Control FX Stop", "Control FX Mode 1", "Control FX Mode 2", "Set Robot Start Position", "Config HW Steer Set", "Config HW Steer Get", "Config HW Steer Save", "Config HW Steer Read", "Config HW Drive Set", "Config HW Drive Get", "Config HW Drive Save", "Config HW Drive Read", "Config HW Specific Set", "Config HW Specific Get", "Config HW Specific Save", "Config HW Specific Read", "Config System Save", "Config System Read", "Config From FP", "Start HW Steer Set", "Default HW Steer Set", "Defalut HW Drive Set"] ("Actions")
        n67 = Unbundle By Name(w331) -> ("ACT Input.Mode"=w333:T29)
        n68 = case shown="\"Turret Auto Angle\"" w333 {
          tunnel: [ENUM_ACT_State."Stopping" ("State") w338 w341 w344 ENUM_ACT_State."Moving Mode 1" ("State")] -> w334
          tunnel: w331 -> [w337 w340 w343 w346 w349]
          tunnel: [w337 w340 w343 w346 w349] -> w332
          tunnel: w330 -> [_ w338 w341 w344 _]
          tunnel: [w335 w339 w342 w345 w347] -> w328
          tunnel: w329 -> [w335 _ _ _ w347]
          frame "STOP" {
          }
          frame "Turret Manual" {
            w339 = T45[] [enum."Control FX Mode 2"] items=["No Action", "Reset Time", "Reset All", "Open HW References", "Control FX Stop", "Control FX Mode 1", "Control FX Mode 2", "Set Robot Start Position", "Config HW Steer Set", "Config HW Steer Get", "Config HW Steer Save", "Config HW Steer Read", "Config HW Drive Set", "Config HW Drive Get", "Config HW Drive Save", "Config HW Drive Read", "Config HW Specific Set", "Config HW Specific Get", "Config HW Specific Save", "Config HW Specific Read", "Config System Save", "Config System Read", "Config From FP", "Start HW Steer Set", "Default HW Steer Set", "Defalut HW Drive Set"] ("Actions")
          }
          frame "Trans Manual Angle Auto" {
            w342 = T45[] [enum."Control FX Mode 2"] items=["No Action", "Reset Time", "Reset All", "Open HW References", "Control FX Stop", "Control FX Mode 1", "Control FX Mode 2", "Set Robot Start Position", "Config HW Steer Set", "Config HW Steer Get", "Config HW Steer Save", "Config HW Steer Read", "Config HW Drive Set", "Config HW Drive Get", "Config HW Drive Save", "Config HW Drive Read", "Config HW Specific Set", "Config HW Specific Get", "Config HW Specific Save", "Config HW Specific Read", "Config System Save", "Config System Read", "Config From FP", "Start HW Steer Set", "Default HW Steer Set", "Defalut HW Drive Set"] ("Actions")
          }
          frame "Turret Auto Angle" {
            w345 = T45[] [enum."Control FX Mode 2"] items=["No Action", "Reset Time", "Reset All", "Open HW References", "Control FX Stop", "Control FX Mode 1", "Control FX Mode 2", "Set Robot Start Position", "Config HW Steer Set", "Config HW Steer Get", "Config HW Steer Save", "Config HW Steer Read", "Config HW Drive Set", "Config HW Drive Get", "Config HW Drive Save", "Config HW Drive Read", "Config HW Specific Set", "Config HW Specific Get", "Config HW Specific Save", "Config HW Specific Read", "Config System Save", "Config System Read", "Config From FP", "Start HW Steer Set", "Default HW Steer Set", "Defalut HW Drive Set"] ("Actions")
          }
          frame "Move" {
          }
        }
      }
      frame "Shutdown" {
        w350 = T45[] [enum."Reset All"] items=["No Action", "Reset Time", "Reset All", "Open HW References", "Control FX Stop", "Control FX Mode 1", "Control FX Mode 2", "Set Robot Start Position", "Config HW Steer Set", "Config HW Steer Get", "Config HW Steer Save", "Config HW Steer Read", "Config HW Drive Set", "Config HW Drive Get", "Config HW Drive Save", "Config HW Drive Read", "Config HW Specific Set", "Config HW Specific Get", "Config HW Specific Save", "Config HW Specific Read", "Config System Save", "Config System Read", "Config From FP", "Start HW Steer Set", "Default HW Steer Set", "Defalut HW Drive Set"] ("Actions")
      }
    }
    n69 = case shown="True" w69 {
      tunnel: w68 -> [_ w355]
      tunnel: [_ w353] -> w67
      frame False {
      }
      frame True {
        n70 = call "Search Unsorted 1D Array.vim"("element"=TRUE, "unsorted 1D array"=w355) -> ("index of element"=w354:i32)  [unwired: 9 in]
        n71 = case shown="..0" w354 {
          tunnel: [w357 w358] -> w353
          frame ..0 {
            w357 = T45[] [enum."Open HW References", enum."Config HW Steer Get", enum."Control FX Mode 1"] items=["No Action", "Reset Time", "Reset All", "Open HW References", "Control FX Stop", "Control FX Mode 1", "Control FX Mode 2", "Set Robot Start Position", "Config HW Steer Set", "Config HW Steer Get", "Config HW Steer Save", "Config HW Steer Read", "Config HW Drive Set", "Config HW Drive Get", "Config HW Drive Save", "Config HW Drive Read", "Config HW Specific Set", "Config HW Specific Get", "Config HW Specific Save", "Config HW Specific Read", "Config System Save", "Config System Read", "Config From FP", "Start HW Steer Set", "Default HW Steer Set", "Defalut HW Drive Set"] ("Actions")
            # "Read Config"
          }
          frame 1.. {
            w358 = T45[] [enum."Config From FP", enum."Config HW Steer Get", enum."Control FX Stop", enum."Control FX Mode 2"] items=["No Action", "Reset Time", "Reset All", "Open HW References", "Control FX Stop", "Control FX Mode 1", "Control FX Mode 2", "Set Robot Start Position", "Config HW Steer Set", "Config HW Steer Get", "Config HW Steer Save", "Config HW Steer Read", "Config HW Drive Set", "Config HW Drive Get", "Config HW Drive Save", "Config HW Drive Read", "Config HW Specific Set", "Config HW Specific Get", "Config HW Specific Save", "Config HW Specific Read", "Config System Save", "Config System Read", "Config From FP", "Start HW Steer Set", "Default HW Steer Set", "Defalut HW Drive Set"] ("Actions")
            # "Updated Config"
          }
        }
      }
    }
    n72 = global write "Global_ACT_Data Out.vi" "ACT_Template_STATE"(w56) -> ()
    n73 = Bundle By Name(cluster=w96, "Previous State"=w56, "State"=w95) -> (w97:T41)
    n74 = Build Array (concatenate)(T42."Open HW Only" ("Action")) -> (w82:T46)  [unwired: 1 in]
    n75 = for {
      tunnel: w82 -> [w129] mode=indexing
      shift-right: [w128] -> w81
      shift-left: w97 -> [w127]
      n76 = case shown="\"Config HW File Read\"" w129 {
        tunnel: w127 -> [w130 w133 w134 w143 w154 w161 w167 w175 w207 w210 w223 w237 w244 w245 w246 w247]
        tunnel: [w130 w132 w134 w147 w155 w162 w168 w176 w208 w209 w222 w238 w244 w245 w246 w247] -> w128
        frame "No Action" {
        }
        frame "Reset Time" {
          n77 = Unbundle By Name(w133) -> ("Current Time"=w131:timestamp)
          n78 = Bundle By Name(cluster=w133, "Start Time"=w131) -> (w132:T41)
        }
        frame "Reset All" {
        }
        frame "Config HW File Read" {
          w135 = FALSE ("Read(f) Write(t)")
          n79 = Unbundle By Name(w143) -> ("Team Folder"=w138:path, "Config HW Drive"=w137:T1, "Config HW Steer"=w146:T8, "Config System"=w140:T17)
          n80 = Unbundle By Name(w143) -> ("Config HW Specific"=w142:T14)
          n81 = call "RWA_File Config.vim"("Read(f) Save(t)"=w135, "Target Folder Folder"=w138, "Any Config"=w140) -> ("Any Config Out"=w139:T17)  [unwired: 4 in, 4 out]
          n82 = call "RWA_File Config.vim"("Read(f) Save(t)"=w135, "Target Folder Folder"=w138, "Any Config"=w146) -> ("Any Config Out"=w145:T8)  [unwired: 4 in, 4 out]
          n83 = call "RWA_File Config.vim"("Read(f) Save(t)"=w135, "Target Folder Folder"=w138, "Any Config"=w142) -> ("Any Config Out"=w141:T14)  [unwired: 4 in, 4 out]
          n84 = call "RWA_File Config.vim"("Read(f) Save(t)"=w135, "Target Folder Folder"=w138, "Any Config"=w137) -> ("Any Config Out"=w136:T1)  [unwired: 4 in, 4 out]
          n85 = Bundle By Name(cluster=w143, "Config HW Drive"=w136, "Config HW Steer"=w145, "Config System"=w139, "Update Display"=TRUE, "Config HW Specific"=w141) -> (w147:T41)
        }
        frame "Control FX Stop" {
          w148 = TRUE ("Read(f) Write(t)")
          n86 = Unbundle By Name(w154) -> ("Team Folder"=w149:path, "HW All Config"=w153:T38, "Config HW Specific"=w151:T14)
          n87 = call "RWA_File Config.vim"("Read(f) Save(t)"=w148, "Target Folder Folder"=w149, "Any Config"=w153) -> ("Any Config Out"=w152:T38)  [unwired: 4 in, 4 out]
          n88 = call "RWA_File Config.vim"("Read(f) Save(t)"=w148, "Target Folder Folder"=w149, "Any Config"=w151) -> ("Any Config Out"=w150:T14)  [unwired: 4 in, 4 out]
          n89 = Bundle By Name(cluster=w154, "HW All Config"=w152, "Config HW Specific"=w150) -> (w155:T41)
        }
        frame "Control FX Mode 1" {
          n90 = Unbundle By Name(w161) -> ("Team Folder"=w158:path, "Config System"=w160:T17)
          n91 = call "RWA_File Config.vim"("Read(f) Save(t)"=FALSE ("Read(f) Write(t)"), "Target Folder Folder"=w158, "Any Config"=w160) -> ("Any Config Out"=w159:T17)  [unwired: 4 in, 4 out]
          n92 = Bundle By Name(cluster=w161, "Config System"=w159, "Update Display"=TRUE) -> (w162:T41)
        }
        frame "Control FX Mode 2" {
          n93 = Unbundle By Name(w167) -> ("Team Folder"=w164:path, "Config System"=w166:T17)
          n94 = call "RWA_File Config.vim"("Read(f) Save(t)"=TRUE ("Read(f) Write(t)"), "Target Folder Folder"=w164, "Any Config"=w166) -> ("Any Config Out"=w165:T17)  [unwired: 4 in, 4 out]
          n95 = Bundle By Name(cluster=w167, "Config System"=w165) -> (w168:T41)
        }
        frame "Set Robot Start Position" {
          n96 = Unbundle By Name(w175) -> ("Config HW Drive"=w182:T1, "Config HW Drive.Drive HW Ver"=w180:u64, "Config HW Steer"=w181:T8, "Config HW Steer.Steer HW Ver"=w177:u64)
          n97 = Unbundle By Name(w175) -> ("Config HW Specific"=w189:T14, "Config HW Specific.Specific HW Ver"=w187:u64)
          n98 = Unbundle By Name(w175) -> ("Current Time"=w197:timestamp)
          n99 = Unbundle By Name(w175) -> ("Config System"=w191:T17, "Config System.System Ver"=w193:u64)
          n100 = call "Date Stamp.vi"("Time"=w197) -> ("U64 Out"=w178:u64)  [unwired: 5 in, 1 out]
          n101 = Not Equal?(x=w191, y="System Config") -> (x != y?=w194:bool)
          n102 = Not Equal?(x="HW Specific Config", y=w189) -> (x != y?=w188:bool)
          n103 = Select(t=w178, s=w194, f=w193) -> (s? t:f=w192:u64)
          n104 = Select(t=w178, s=w188, f=w187) -> (s? t:f=w185:u64)
          n105 = Not Equal?(x="Config Steer", y=w181) -> (x != y?=w179:bool)
          n106 = Bundle By Name(cluster="System Config", "System Ver"=w192) -> (w196:T17)
          n107 = Not Equal?(x="Config Drive", y=w182) -> (x != y?=w190:bool)
          n108 = Select(t=w178, s=w179, f=w177) -> (s? t:f=w169:u64)
          n109 = Bundle By Name(cluster="Config Steer", "Steer HW Ver"=w169) -> (w170:T8)
          n110 = Bundle By Name(cluster="HW Specific Config", "Specific HW Ver"=w185) -> (w184:T14)
          n111 = Select(t=w178, s=w190, f=w180) -> (s? t:f=w173:u64)
          n112 = Bundle By Name(cluster="Config Drive", "Drive HW Ver"=w173) -> (w172:T1)
          n113 = Bundle By Name(cluster=w175, "Config HW Drive"=w172, "Config HW Steer"=w170, "Update Display"=TRUE, "Config System"=w196, "Config HW Specific"=w184) -> (w176:T41)
        }
        frame "Config HW All Get" {
          n114 = Unbundle By Name(w207) -> ("Drive Refs"=w201:T33[], "Steer Refs"=w200:T33[], "HW All Config"=w204:T38, "CAN Timeout"=w205:u32)
          n115 = Index Array(array=w200) -> (element=w198:T33)  [unwired: 1 in]
          n116 = Index Array(array=w201) -> (element=w199:T33)  [unwired: 1 in]
          n117 = call "Config HW Extract.vi"("Get(f) Set(t)"=FALSE, "Send Cmd Timout(ms)"=w205, "Drive Refs"=w199, "HW Config"=w204, "Steer Refs"=w198) -> ("HW Config Out"=w203:T47)  [unwired: 3 in, 3 out]
          n118 = Bundle By Name(cluster=w207, "HW All Config"=w203, "Update Display"=TRUE) -> (w208:T41)
        }
        frame "Config HW Set Steer" {
          n119 = in-place {
            n120 = in-place-cluster #1(w210) -> ("HW All Config.Steer"=w212:T8, "Steer Refs"=w214:T33[])
            n121 = for {
              tunnel: w214 -> [w221] mode=indexing
              tunnel: [w220] -> w213 mode=indexing
              shift-right: [w218] -> w211
              shift-left: w212 -> [w219]
              n122 = call "Config Steer Module Get-Set.vi"("Start With Default"=FALSE, "Get(f) Set(t)"=TRUE, "Set Steer Values"=w219, "Send Cmd Timout(ms)"=u32 300, "Steer Refs"=w221) -> ("Steer Refs Out"=w220:T33, "Steer Config Out"=w218:T8)  [unwired: 3 in, 2 out]
            }
            n123 = in-place-cluster #1("HW All Config.Steer"=w211, "Steer Refs"=w213) -> (w209:T41)
          }
        }
        frame "Config HW Set Drive" {
          n124 = in-place {
            n125 = in-place-cluster #2(w223) -> ("HW All Config.Drive"=w225:T1, "Drive Refs"=w227:T33[])
            n126 = for {
              tunnel: w227 -> [w233] mode=indexing
              tunnel: [w232] -> w226 mode=indexing
              shift-right: [w230] -> w224
              shift-left: w225 -> [w231]
              n127 = call "Config Drive Module Get-Set.vi"("Start with Default"=FALSE ("Start With Default"), "Get(f) Set(t)"=TRUE, "Set Drive Config"=w231, "Drive Refs"=w233) -> ("Drive Refs Out"=w232:T33, "Drive Config Out"=w230:T1)  [unwired: 5 in, 1 out]
            }
            n128 = in-place-cluster #2("HW All Config.Drive"=w224, "Drive Refs"=w226) -> (w222:T41)
          }
        }
        frame "Open HW Only" {
          n129 = Unbundle By Name(w237) -> ("Config HW Specific.Specific Data"=w236:T15[])
          n130 = for {
            tunnel: w236 -> [w243] mode=indexing
            tunnel: [w241] -> w235 mode=indexing
            tunnel: [w239] -> w234 mode=indexing
            n131 = Unbundle By Name(w243) -> ("Drive ID"=w242:u8, "Steer ID"=w240:u8)  [unwired: 1 out]
            n132 = call <vilib>:"CTRE_Phoenix_TalonSRX_Open.vi"("Device Number"=w240) -> ("PhoenixMotorControlDevRef"=w239:T33)  [unwired: 9 in, 1 out]
            n133 = call <vilib>:"Spark MAX Open.vi"("Device Number"=w242) -> ("MotorControlDeviceRef"=w241:T33)  [unwired: 9 in, 1 out]
          }
          n134 = Bundle By Name(cluster=w237, "Steer Refs"=w235, "Drive Refs"=w234) -> (w238:T41)
        }
        frame "Set Robot Start Position" {
          # "#Fix"
        }
        frame "Control FX Stop" {
          # "#Fix"
        }
        frame "Control FX Mode 1" {
          # "#Fix"
        }
        frame "Control FX Mode 2" {
          # "#Fix"
        }
      }
    }
    n135 = Unbundle By Name(w81) -> ("Config System"=w36:T17, "Config HW Drive"=w37:T1, "Config HW Steer"=w78:T8, "Update Display"=w79:bool, "Config System"=w61:T17, "Config HW Specific"=w44:T14)
    n136 = Unbundle By Name(w81) -> ("State"=w77:T40)
    n137 = Unbundle By Name(w81) -> ("Cycle Time(S)"=w83:dbl)
    "Cycle Time (S)" <- w83
    n138 = Unbundle By Name(w81) -> ("ACT Input"=→"CMD":T28, "HW Out"=w75:T23, "System Output"=w66:T22)
    "HW Output" <- w75
    "System Config" <- w66
    n139 = case shown="\"Startup\", \"Configuring\"" w77 {
      frame "Startup", "Configuring" {
        # "#Fix"
      }
      frame Default {
      }
    }
    n140 = case shown="True" w79 {
      tunnel: w78 -> [_ w361]
      tunnel: w61 -> [_ w363]
      tunnel: w44 -> [_ w362]
      tunnel: w37 -> [_ w360]
      tunnel: w36 -> [_ w359]
      frame False {
      }
      frame True {
        n141 = local write "System Config"(w363) -> ()
        n142 = local write "HW Specific Config"(w362) -> ()
        n143 = local write "Config Steer"(w361) -> ()
        n144 = local write "System Config"(w359) -> ()
        n145 = local write "Config Drive"(w360) -> ()
      }
    }
    n146 = global write "Global_ACT_Data Out.vi" "ACT_Template_System Output"(w66) -> ()
    n147 = global write "Global_ACT_Data Out.vi" "ACT_Template_HW Output"(w75) -> ()
    n148 = global write "Global_ACT_Data Out.vi" "ACT_Template_CycleTime(S)"(w83) -> ()
    n149 = Bundle By Name(cluster=w81, "Update Display"=FALSE) -> (w84:T41)
  }
  n150 = flat-sequence {
    frame #0 {
      (unwired) ENUM_ACT_Action."Open HW Only" ("Action")
      (unwired) ENUM_ACT_State."Startup" ("State")
      (unwired) ENUM_ACT_Action."Config HW All Get" ("Action")
      # "State LIST"
      # "Action LIST"
    }
  }
  n151 = Unbundle By Name(w24) -> ("Steer Refs"=w21:T33[], "Drive Refs"=w8:T33[])
  n152 = for {
    tunnel: w21 -> [w365] mode=indexing
    tunnel: w8 -> [w364] mode=indexing
    n153 = call <vilib>:"WPI_MotorControlDisable.vi"("MotorControlDevRef"=w364) -> ()  [unwired: 9 in, 2 out]
    n154 = call <vilib>:"WPI_MotorControlDisable.vi"("MotorControlDevRef"=w365) -> ()  [unwired: 9 in, 2 out]
  }
